vi "init.vi"(3 "Container State":T4 caption="État du conteneur", 4 "Previous State":variant caption="État précédent", 5 "Previous Version":T3 caption="Version précédente") -> (2 "Current State":T1 caption="État actuel")   [LabVIEW 2013, in "slot.xctl"]
uses:
  slot.xctl
  state.ctl
  slot-use.ctl
  <vilib>/_xctls/Container State.ctl
  <vilib>/_xctls/Version.ctl
  <vilib>/_xctls/XControlSupport.lvlib
panel:
  in  "Default Indicator State":T1 caption="État de l'indicateur par défaut"
  in  "Default Control State":T1 caption="État de la commande par défaut"
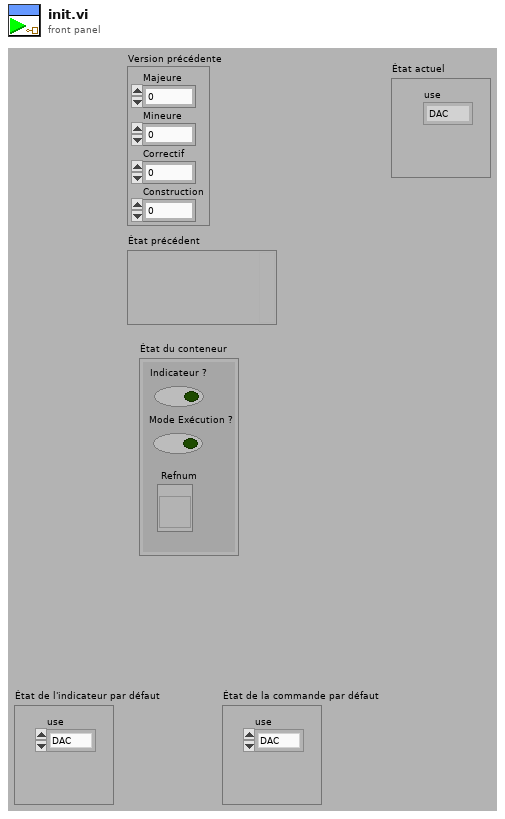
[diagram p1: front panel]
types:
  T1 = typedef "slot.xctl/state.ctl" = cluster{"use":T2}
  T2 = typedef "slot-use.ctl" = enum8{"DAC", "timing", "triggers", "jump"}
  T3 = typedef "XControlSupport.lvlib/Version.ctl" = cluster{"Major":u16, "Minor":u16, "Fix":u16, "Build":u16}
  T4 = typedef "XControlSupport.lvlib/Container State.ctl" = cluster{"Indicator?":bool, "Run Mode?":bool, " Refnum":refnum<vi>}
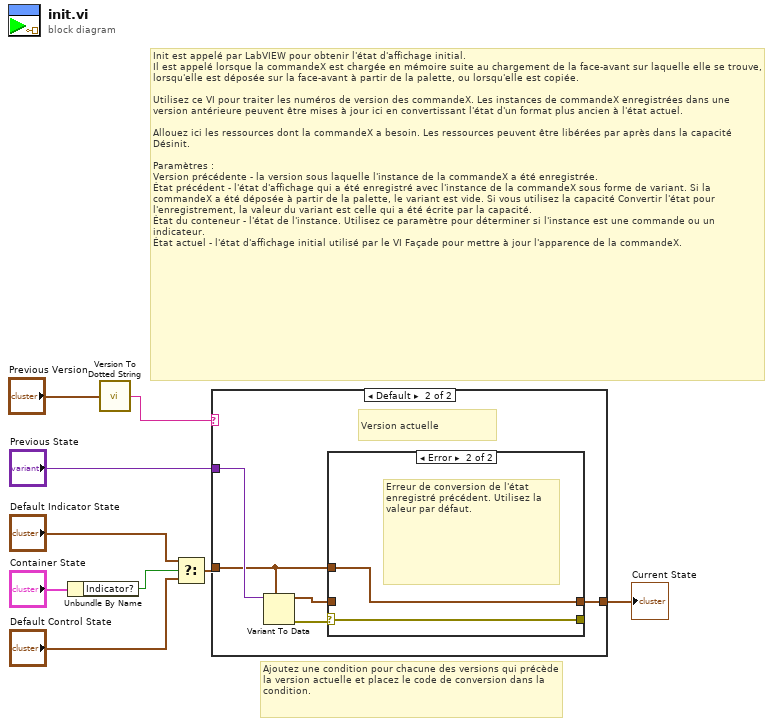
[diagram p0: block diagram]
diagram:
  # "Ajoutez une condition pour chacune des versions qui précède la version actuelle et placez le code de conversion dans la condition."
  # "Init est appelé par LabVIEW pour obtenir l'état d'affichage initial.\nIl est appelé lorsque la commandeX est chargée en mémoire suite au chargement de la face-avant sur laquelle elle se trouve, lorsqu'elle est déposée sur la face-avant à partir de la palette, ou lorsqu'elle est copiée.\n\nUtilisez ce VI pour traiter les numéros de version des commandeX. Les instances de commandeX enregistrées dans une version antérieure peuvent être mises à jour ici en convertissant l'état d'un format plus ancien à l'état actuel.\n\nAllouez ici les ressources dont la commandeX a besoin. Les ressources peuvent être libérées par après dans la capacité Désinit.\n\nParamètres :\nVersion précédente - la version sous laquelle l'instance de la commandeX a été enregistrée.\nÉtat précédent - l'état d'affichage qui a été enregistré avec l'instance de la commandeX sous forme de variant. Si la commandeX a été déposée à partir de la palette, le variant est vide. Si vous utilisez la capacité Convertir l'état pour l'enregistrement, la valeur du variant est celle qui a été écrite par la capacité. \nÉtat du conteneur - l'état de l'instance. Utilisez ce paramètre pour déterminer si l'instance est une commande ou un indicateur.\nÉtat actuel - l'état d'affichage initial utilisé par le VI Façade pour mettre à jour l'apparence de la commandeX."
  n1 = Unbundle By Name("Container State") -> ("Indicator?"=w4:bool)
  n2 = call <vilib>:"Version To Dotted String.vi"("Version"="Previous Version") -> ("String Version"=w1:string)
  n3 = Select(t="Default Indicator State", s=w4, f="Default Control State") -> (s? t:f=w3:T1)
  n4 = case shown="Default" w1 {
    tunnel: "Previous State" -> [_ w15]
    tunnel: [w10 w11] -> w8
    tunnel: w3 -> [w10 w12]
    frame "0.0.0.0" {
      # "Nouvelle création ; utilisez l'état par défaut"
    }
    frame Default {
      # "Version actuelle"
      n5 = Variant To Data(type=w12, Variant=w15) -> (data=w13:T1, error out=w14:errorcluster)  [unwired: 1 in]
      n6 = case shown="Error" w14 {
        selector: w14 -> [w17 w18]
        tunnel: w13 -> [w16 _]
        tunnel: [w16 w19] -> w11
        tunnel: w12 -> [_ w19]
        tunnel: [w17 w18] -> _
        frame No Error {
        }
        frame Error {
          # "Erreur de conversion de l'état\nenregistré précédent. Utilisez la valeur par défaut."
        }
      }
    }
  }
  "Current State" <- w8
